vi "ReversedEngineering_MergeEdges.vi"(0 "EdgesCreated":refnum<class "AbstractEdge.lvclass">[](array[class]), 1 "EdgesToMerge":refnum<class "AbstractEdge.lvclass">[](array[class])) -> (14 "EdgesOut":refnum<class "AbstractEdge.lvclass">[](array[class]))   [LabVIEW 2016]
uses:
  <resource>/Framework/Providers/Open_GDS/UML/AbstractEdge_class/AbstractEdge.lvclass
  <resource>/Framework/Providers/Open_GDS/UML/ClassRelationshipEdge_class/ClassRelationshipEdge.lvclass
  C:/Program Files (x86)/National Instruments/LabVIEW 2016/resource/Framework/Providers/Open_GDS/UML/AbstractEdge_class/AbstractEdge.lvclass
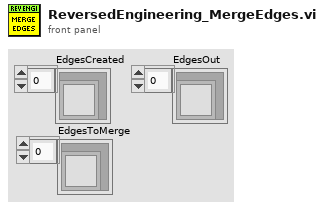
[diagram p1: front panel]
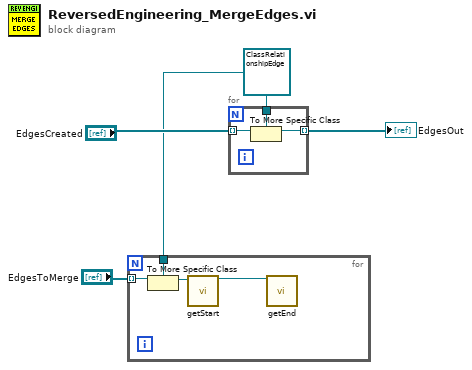
[diagram p0: block diagram]
diagram:
  w1 = refnum<class "ClassRelationshipEdge.lvclass"> refnum ("reference")
  n1 = for {
    tunnel: "EdgesToMerge" -> [w7] mode=indexing
    tunnel: w1 -> [w5]
    n2 = To More Specific Class(target class=w5, reference=w7) -> (specific class reference=w6:refnum<class "ClassRelationshipEdge.lvclass">)  [unwired: 1 in, 1 out]
    n3 = call-dynamic "getStart.vi"("reference"=w6) -> ("reference out"=w8:refnum<class "ClassRelationshipEdge.lvclass">)  [unwired: 15 in, 3 out]
    n4 = call-dynamic "getEnd.vi"("reference"=w8) -> ()  [unwired: 15 in, 4 out]
  }
  n5 = for {
    tunnel: w1 -> [w11]
    tunnel: "EdgesCreated" -> [w10] mode=indexing
    tunnel: [w9] -> w3 mode=indexing
    n6 = To More Specific Class(target class=w11, reference=w10) -> (specific class reference=w9:refnum<class "ClassRelationshipEdge.lvclass">)  [unwired: 1 in, 1 out]
  }
  "EdgesOut" <- w3
